vi "Check Unique and Valid Mapping.vi"(8 "error in (no error)":errorcluster, 9 "Destination Path":string, 10 "Source Path":string, 11 "SDF Ref":refnum<k24>) -> (0 "error out":errorcluster, 2 "Mapping Error":T1)   [LabVIEW 2016, in "System Mapping Tool.lvlib"]
uses:
  System Mapping Tool.lvlib
  NationalInstruments.VeriStand.SystemDefinitionAPI
  TypeDefs/Mapping Error Cluster.ctl
  TypeDefs/Mapping Error.ctl
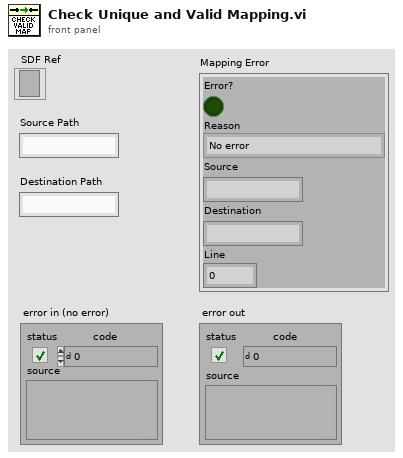
[diagram p1: front panel]
types:
  T1 = typedef "System Mapping Tool.lvlib/Mapping Error Cluster.ctl" = cluster{"Error?":bool, "Reason":T2, "Source":string, "Destination":string, "Line":i32}
  T2 = typedef "System Mapping Tool.lvlib/Mapping Error.ctl" = enum16{"No error", "Channels already mapped", "Source is not valid", "Destination is not valid", "Destination already mapped", "Destination mapped twice"}
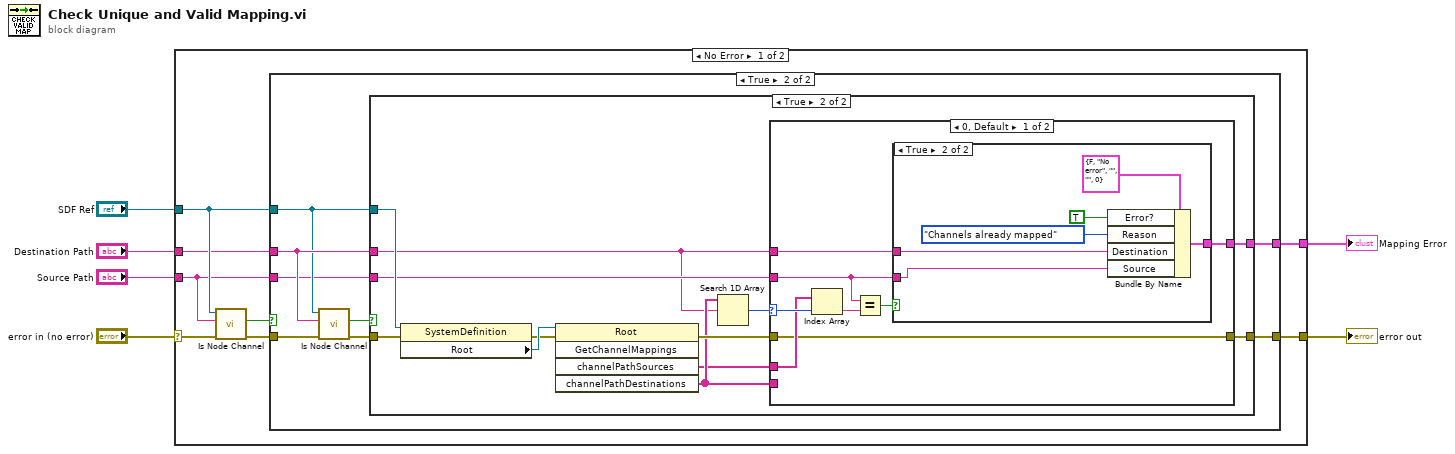
[diagram p0: block diagram]
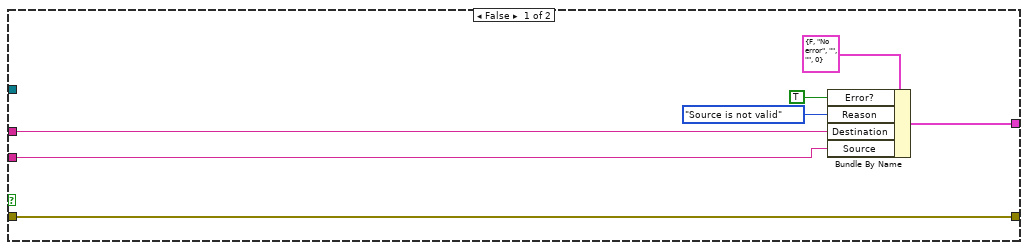
[diagram p2: hidden frame]
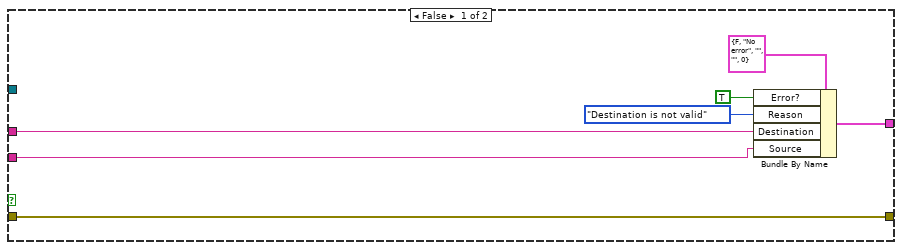
[diagram p3: hidden frame]
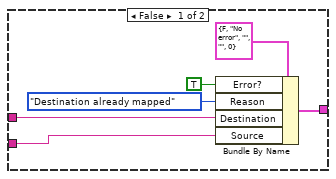
[diagram p4: hidden frame]
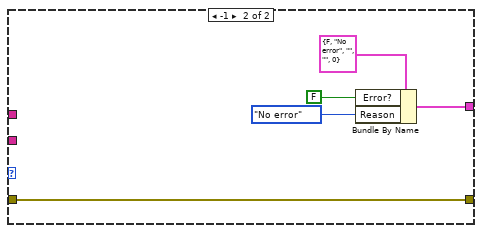
[diagram p5: hidden frame]
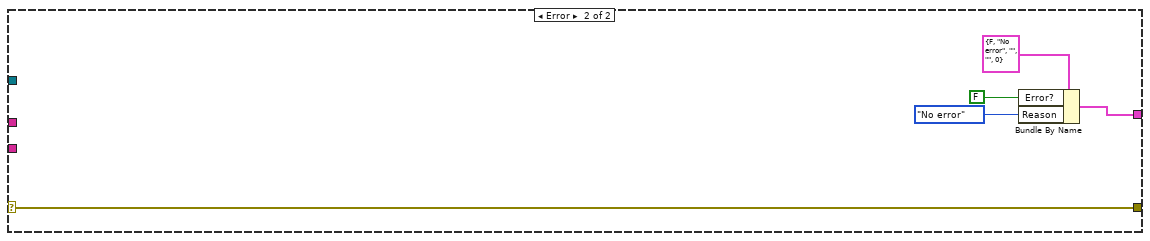
[diagram p6: hidden frame]
diagram:
  n1 = case shown="No Error" "error in (no error)" {
    selector: "error in (no error)" -> [w14 w78]
    tunnel: [w8 w78] -> w5
    tunnel: "Destination Path" -> [w11 _]
    tunnel: "Source Path" -> [w9 _]
    tunnel: "SDF Ref" -> [w12 _]
    tunnel: [w7 w74] -> w1
    frame No Error {
      n2 = call "Is Node Channel.vi"("error in (no error)"=w14, "Node Path"=w9, "SDF Ref"=w12) -> ("error out"=w13:errorcluster, "Is Channel?"=w10:bool)  [unwired: 7 in]
      n3 = case shown="True" w10 {
        tunnel: w13 -> [w21 w29]
        tunnel: w12 -> [_ w24]
        tunnel: w11 -> [w15 w25]
        tunnel: w9 -> [w16 w23]
        tunnel: [w21 w26] -> w8
        tunnel: [w17 w22] -> w7
        frame False {
          n4 = Bundle By Name(cluster=T1 {"Error?"=FALSE, "Reason"=enum."No error", "Source"="", "Destination"="", "Line"=0} ("Mapping Error"), "Error?"=TRUE, "Reason"=Mapping_Error."Source is not valid", "Destination"=w15, "Source"=w16) -> (w17:T1)
        }
        frame True {
          n5 = call "Is Node Channel.vi"("error in (no error)"=w29, "Node Path"=w25, "SDF Ref"=w24) -> ("error out"=w27:errorcluster, "Is Channel?"=w28:bool)  [unwired: 7 in]
          n6 = case shown="True" w28 {
            tunnel: w27 -> [w36 w48]
            tunnel: [w36 w43] -> w26
            tunnel: w25 -> [w32 w38]
            tunnel: w24 -> [_ w47]
            tunnel: w23 -> [w30 w39]
            tunnel: [w31 w37] -> w22
            frame False {
              n7 = Bundle By Name(cluster=T1 {"Error?"=FALSE, "Reason"=enum."No error", "Source"="", "Destination"="", "Line"=0} ("Mapping Error"), "Error?"=TRUE, "Reason"=Mapping_Error."Destination is not valid", "Destination"=w32, "Source"=w30) -> (w31:T1)
            }
            frame True {
              n8 = property class="SystemDefinition"(reference=w47, error in=w48) -> (error out=w45:errorcluster, "Root"=w46:refnum<k24>)  [unwired: 1 out]
              n9 = invoke class="Root" method="GetChannelMappings"(reference=w46, error in=w45) -> (error out=w42:errorcluster, "channelPathSources"=w40:string[], "channelPathDestinations"=w41:string[])  [unwired: 3 in, 2 out]
              n10 = Search 1D Array(1D array=w41, element=w38) -> (index of element=w44:i32)  [unwired: 1 in]
              n11 = case shown="0, Default" w44 {
                selector: w44 -> [w56 _]
                tunnel: [w53 w73] -> w43
                tunnel: w42 -> [w53 w73]
                tunnel: w41 -> [_ _]
                tunnel: w40 -> [w55 _]
                tunnel: w39 -> [w50 _]
                tunnel: w38 -> [w51 _]
                tunnel: [w49 w69] -> w37
                frame 0, Default {
                  n12 = Index Array(array=w55, index=w56) -> (element=w54:string)
                  n13 = Equal?(x=w50, y=w54) -> (x = y?=w52:bool)
                  n14 = case shown="True" w52 {
                    tunnel: w51 -> [w58 w63]
                    tunnel: w50 -> [w57 w64]
                    tunnel: [w59 w65] -> w49
                    frame False {
                      n15 = Bundle By Name(cluster=T1 {"Error?"=FALSE, "Reason"=enum."No error", "Source"="", "Destination"="", "Line"=0} ("Mapping Error"), "Error?"=TRUE, "Reason"=Mapping_Error."Destination already mapped", "Destination"=w58, "Source"=w57) -> (w59:T1)
                    }
                    frame True {
                      n16 = Bundle By Name(cluster=T1 {"Error?"=FALSE, "Reason"=enum."No error", "Source"="", "Destination"="", "Line"=0} ("Mapping Error"), "Error?"=TRUE, "Reason"=Mapping_Error."Channels already mapped", "Destination"=w63, "Source"=w64) -> (w65:T1)
                    }
                  }
                }
                frame -1 {
                  n17 = Bundle By Name(cluster=T1 {"Error?"=FALSE, "Reason"=enum."No error", "Source"="", "Destination"="", "Line"=0} ("Mapping Error"), "Error?"=FALSE, "Reason"=Mapping_Error."No error") -> (w69:T1)
                }
              }
            }
          }
        }
      }
    }
    frame Error {
      n18 = Bundle By Name(cluster=T1 {"Error?"=FALSE, "Reason"=enum."No error", "Source"="", "Destination"="", "Line"=0} ("Mapping Error"), "Error?"=FALSE, "Reason"=Mapping_Error."No error") -> (w74:T1)
    }
  }
  "error out" <- w5
  "Mapping Error" <- w1
